vi "CLSUIP_GetUnlockPrompt.vi"(1 "VIRetooler":refnum<class "VIRetooler.lvclass">) -> (0 "localized prompt 2":string="%s is password-protected.  You must enter the password to create a VI for override using this VI as a template.")   [LabVIEW 2021, in "MemberVICreation.lvlib" / "VIRetooler.lvclass"]
uses:
  <resource>/Framework/Providers/LVClassLibrary/NewAccessors/VIRetooler/VIRetooler.lvclass
panel:
  in  "localized prompt":string="%s is password-protected.  You must enter the password to create a VI for override using this VI as a template."
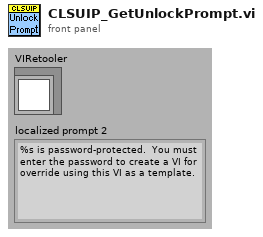
[diagram p1: front panel]
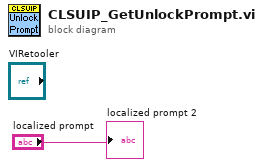
[diagram p0: block diagram]
diagram:
  "localized prompt 2" <- "localized prompt"
